vi "Get_VITerminalNamesandConnum.vi"(11 "VI Path":path) -> (1 "Connum":i32[](array[numeric]), 2 "VI Terminal Names":string[](array[string]))   [LabVIEW 2020]
uses:
  <vilib>/Utility/VariantDataType/VariantType.lvlib
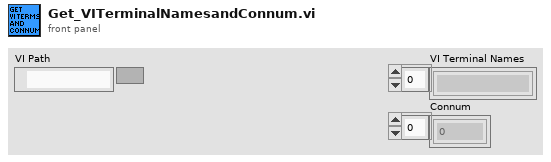
[diagram p1: front panel]
types:
  T1 = typedef "VariantType.lvlib/VIInfo.ctl" = cluster{"Data1":i16, "Data2":i16, "Flags":u32[], "Modification Date":timestamp, "Asynchronous":bool, "NonFunctional":bool, "Subroutine":bool, "SubSystem":bool}
  T2 = typedef "VariantType.lvlib/Type.ctl" = enum8{"Invalid Type", "Void", "I8", "I16", "I32", "I64", "U8", "U16", "U32", "U64", "Single Float", "Double Float", "Extended Float", "Single Complex", "Double Complex", "Extended Complex", "Enum U8", "Enum U16", "Enum U32", "Enum U64", "Single Float With Unit", "Double Float With Unit", "Extended Float With Unit", "Single Complex with Unit", "Double Complex with Unit", "Extended Complex with Unit", "Boolean", "String", "Path", "Picture", "Tag", "Array", "Cluster", "Variant", "LV Variant", "Waveform", "Timestamp", "Digital Waveform", "Digital Data", "ExpressData", "Refnum", "External Data", "VI", "Poly VI", "LabVIEW Class Instance", "Fixed Point"}
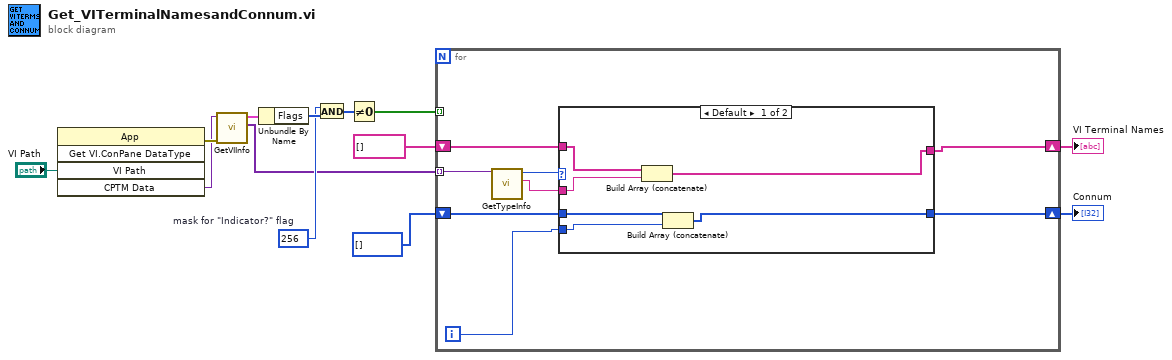
[diagram p0: block diagram]
diagram:
  w8 = i16 256  # mask for "Indicator?" flag
  n1 = invoke class="App" method="Get VI.ConPane DataType"("VI Path"="VI Path") -> (error out=w12:errorcluster, "CPTM Data"=w11:variant)  [unwired: 4 in, 3 out]
  n2 = call <vilib>:"GetVIInfo.vi"("error in (no error)"=w12, "Variant"=w11) -> ("VI Terminal Types"=w5:variant[], "VI Info"=w10:T1)  [unwired: 8 out]
  n3 = Unbundle By Name(w10) -> ("Flags"=w9:u32[])
  n4 = And(x=w8, y=w9) -> (x .and. y?=w7:u32[])
  n5 = Not Equal To 0?(x=w7) -> (x != 0?=w6:bool[])
  n6 = for {
    tunnel: w6 -> [_] mode=indexing
    tunnel: w5 -> [w21] mode=indexing
    shift-right: [w14] -> w2
    shift-left: string[] [] ("appended array") -> [w18]
    shift-right: [w15] -> w1
    shift-left: i32[] [] ("appended array") -> [w16]
    i -> [w17]
    n7 = call <vilib>:"GetTypeInfo.vi"("Variant"=w21) -> ("Name"=w19:string, "Type Enum"=w20:T2)  [unwired: 1 in, 8 out]
    n8 = case shown="Default" w20 {
      tunnel: w19 -> [w26 _]
      tunnel: w18 -> [w27 w29]
      tunnel: w17 -> [w23 _]
      tunnel: w16 -> [w24 w28]
      tunnel: [w22 w28] -> w15
      tunnel: [w25 w29] -> w14
      frame Default {
        n9 = Build Array (concatenate)(w27, w26) -> (w25:string[])
        n10 = Build Array (concatenate)(w24, w23) -> (w22:i32[])
      }
      frame "Void" {
      }
    }
  }
  "VI Terminal Names" <- w2
  "Connum" <- w1
